vi "TimerSubVI.vi"(2 "s":bool) -> (10 "t":dbl)   [LabVIEW 2022 SP3]
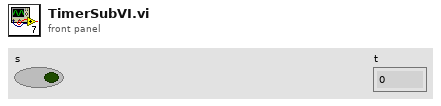
[diagram p1: front panel]
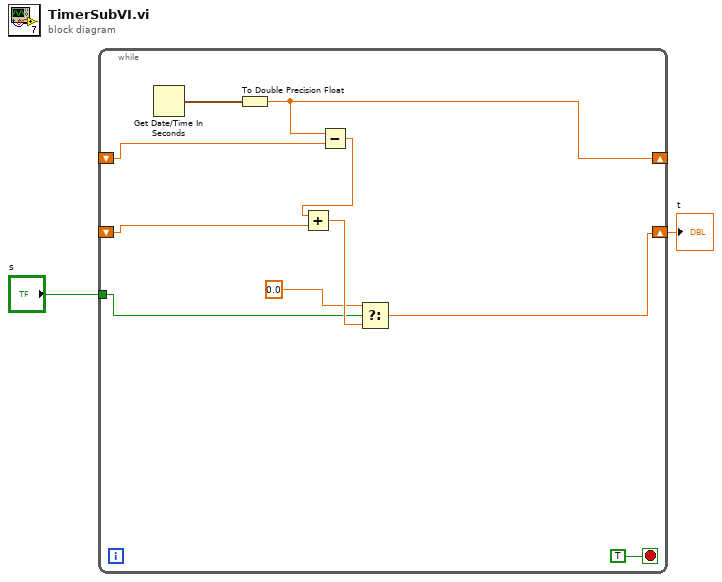
[diagram p0: block diagram]
diagram:
  n1 = while {
    tunnel: "s" -> [w4]
    shift-right: [w9] -> _
    shift-left: _ -> [w10]
    shift-right: [w6] -> w1
    shift-left: _ -> [w5]
    stop <- TRUE stop-if-true
    n2 = Get Date/Time In Seconds() -> (seconds since 1Jan1904=w11:timestamp)
    n3 = To Double Precision Float(number=w11) -> (double precision float=w9:dbl)
    n4 = Subtract(x=w9, y=w10) -> (x-y=w8:dbl)
    n5 = Add(x=w8, y=w5) -> (x+y=w7:dbl)
    n6 = Select(t=0.0, s=w4, f=w7) -> (s? t:f=w6:dbl)
  }
  "t" <- w1
